vi "state_machine_aerial_robot_version_2.vi"() -> ()   [LabVIEW 2019]
uses:
  Control 1.ctl
  <vilib>/myRIO/Instrument Drivers/Onboard IO/DIO/typedefs/DIO Reference.ctl
  <vilib>/myRIO/Common/Instrument Driver Framework/Utilities/typedefs/myRIO Generic Hardware Reference.ctl
  <vilib>/myRIO/Common/Instrument Driver Framework/Utilities/typedefs/Hardware Version Enum.ctl
  <vilib>/myRIO/Common/Instrument Driver Framework/Utilities/typedefs/myRIO v1.0 Reference.ctl
  <vilib>/myRIO/Common/Instrument Driver Framework/Utilities/typedefs/Generic FPGA Reference.ctl
  <vilib>/myRIO/Common/Instrument Driver Framework/myRIO v1.0/DIO/typedefs/DIO Channels List.ctl
  <vilib>/myRIO/Common/Instrument Driver Framework/myRIO v1.0/DIO/typedefs/DIO Channels Enum.ctl
  <vilib>/userdefined/High Color/nirio_resource_hc.ctl
  <vilib>/myRIO/Common/Instrument Driver Framework/Utilities/vis/Is FPGA Ref Available.vi
  <vilib>/myRIO/Common/Instrument Driver Framework/myRIO v1.0/DIO/vis/myRIO v1.1 Open DIO.vi
  <vilib>/myRIO/Instrument Drivers/Onboard IO/DIO/vis/Write.vi
  <vilib>/myRIO/Common/Instrument Driver Framework/Utilities/vis/Validate Channels.vi
  <vilib>/myRIO/Common/Instrument Driver Framework/myRIO v1.0/DIO/vis/myRIO v1.0 Reserve DIO.vi
  <vilib>/myRIO/Common/Instrument Driver Framework/myRIO v1.0/Resource Manager/vis/myRIO v1.0 Reserve Channel List.vi
  <vilib>/myRIO/Common/Instrument Driver Framework/myRIO v1.0/DIO/vis/myRIO v1.0 Build MUX Configuration DIO.vi
  <vilib>/myRIO/Common/Instrument Driver Framework/myRIO v1.0/Resource Manager/vis/myRIO v1.0 Reserve Channel.vi
  <vilib>/myRIO/Common/Instrument Driver Framework/myRIO v1.0/Resource Manager/vis/myRIO v1.0 Unreserve Channel.vi
  <vilib>/myRIO/Common/Instrument Driver Framework/myRIO v1.0/Resource Manager/vis/myRIO v1.0 Create Configuration List.vi
  <vilib>/myRIO/Common/Instrument Driver Framework/myRIO v1.0/Resource Manager/vis/myRIO v1.0 Build Mutex Name.vi
  <vilib>/Utility/VariantDataType/GetNumericInfo.vi
  <vilib>/Utility/error.llb/Error Cluster From Error Code.vi
  <vilib>/myRIO/Common/Instrument Driver Framework/myRIO v1.0/myRIO v1.1 Open.vi
  <vilib>/myRIO/Common/Instrument Driver Framework/Utilities/vis/IO Manager.vi
  <vilib>/myRIO/Common/Instrument Driver Framework/Utilities/vis/Configuration Manager.vi
  <vilib>/myRIO/Common/Instrument Driver Framework/myRIO v1.0/Resource Manager/vis/myRIO v1.0 Configure IO.vi
  <vilib>/myRIO/Common/Instrument Driver Framework/myRIO v1.0/myRIO v1.0 Close.vi
  <vilib>/myRIO/Common/Instrument Driver Framework/myRIO v1.0/DIO/vis/myRIO v1.0 Write DIO.vi
  <vilib>/myRIO/Express VI/Onboard IO/DO/DO Express VI.xnode
  <vilib>/myRIO/Instrument Drivers/Onboard IO/DIO/vis/myRIO DIO Open.xnode
  <vilib>/myRIO/Express VI/Onboard Devices/LED/LED Express VI.xnode
  <vilib>/myRIO/Instrument Drivers/Onboard IO/DIO/DIO.lvlib
panel:
  out "Sensor_inserted?":bool
  out "drone_lifting?":bool
  out "measurement_number":i32
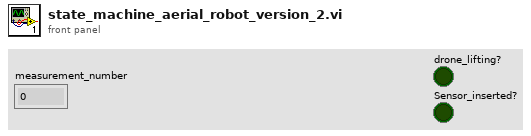
[diagram p1: front panel]
types:
  T1 = typedef "Control 1.ctl" = enum16{"Default", "state 1", "state 2", "state 3", "state 4", "state 5"}
  T2 = typedef "DIO.lvlib/DIO Reference.ctl" = cluster{"myRIO Reference":T3, "DIO Channels List":T7}
  T3 = typedef "myRIO Generic Hardware Reference.ctl" = cluster{"myRIO Model":T4, "myRIO Hardware Reference":T5}
  T4 = typedef "Hardware Version Enum.ctl" = enum16{"Unknown", "myRIO-1900", "myRIO-1950", "roboRIO", "NI ELVIS RIO CM", "ELVIS III"}
  T5 = typedef "myRIO v1.0 Reference.ctl" = cluster{"Generic FPGA Reference":T6, "Allow multiple opens":bool}
  T6 = typedef "Generic FPGA Reference.ctl" = refnum<k20>
  T7 = typedef "DIO Channels List.ctl" = T8[]
  T8 = typedef "DIO Channels Enum.ctl" = enum16{"Not Connected", "C/DIO0", "C/DIO1", "C/DIO2", "C/DIO3", "C/DIO4", "C/DIO5", "C/DIO6", "C/DIO7", "A/DIO0", "A/DIO1", "A/DIO2", "A/DIO3", "A/DIO4", "A/DIO5", "A/DIO6", "A/DIO7", "A/DIO8", "A/DIO9", "A/DIO10", "A/DIO11", "A/DIO12", "A/DIO13", "A/DIO14", "A/DIO15", "A/DIO16", "A/DIO17", "A/DIO18", "A/DIO19", "B/DIO0", "B/DIO1", "B/DIO2", "B/DIO3", "B/DIO4", "B/DIO5", "B/DIO6", "B/DIO7", "B/DIO8", "B/DIO9", "B/DIO10", "B/DIO11", "B/DIO12", "B/DIO13", "B/DIO14", "B/DIO15", "B/DIO16", "B/DIO17", "B/DIO18", "B/DIO19", "LED0", "LED1", "LED2", "LED3", "Button0", "DIO/DIO0", "DIO/DIO1", "DIO/DIO2", "DIO/DIO3", "DIO/DIO4", "DIO/DIO5", "DIO/DIO6", "DIO/DIO7", "DIO/DIO8", "DIO/DIO9", "SPI/CS0", "SPI/CS1", "SPI/CS2", "SPI/CS3", "LED RADIO (Green)", "LED RADIO (Red)", "LED COMM (Green)", "LED COMM (Red)", "LED MODE (Green)", "LED MODE (Red)"}
  T9 = typedef "nirio_resource_hc.ctl" = tag
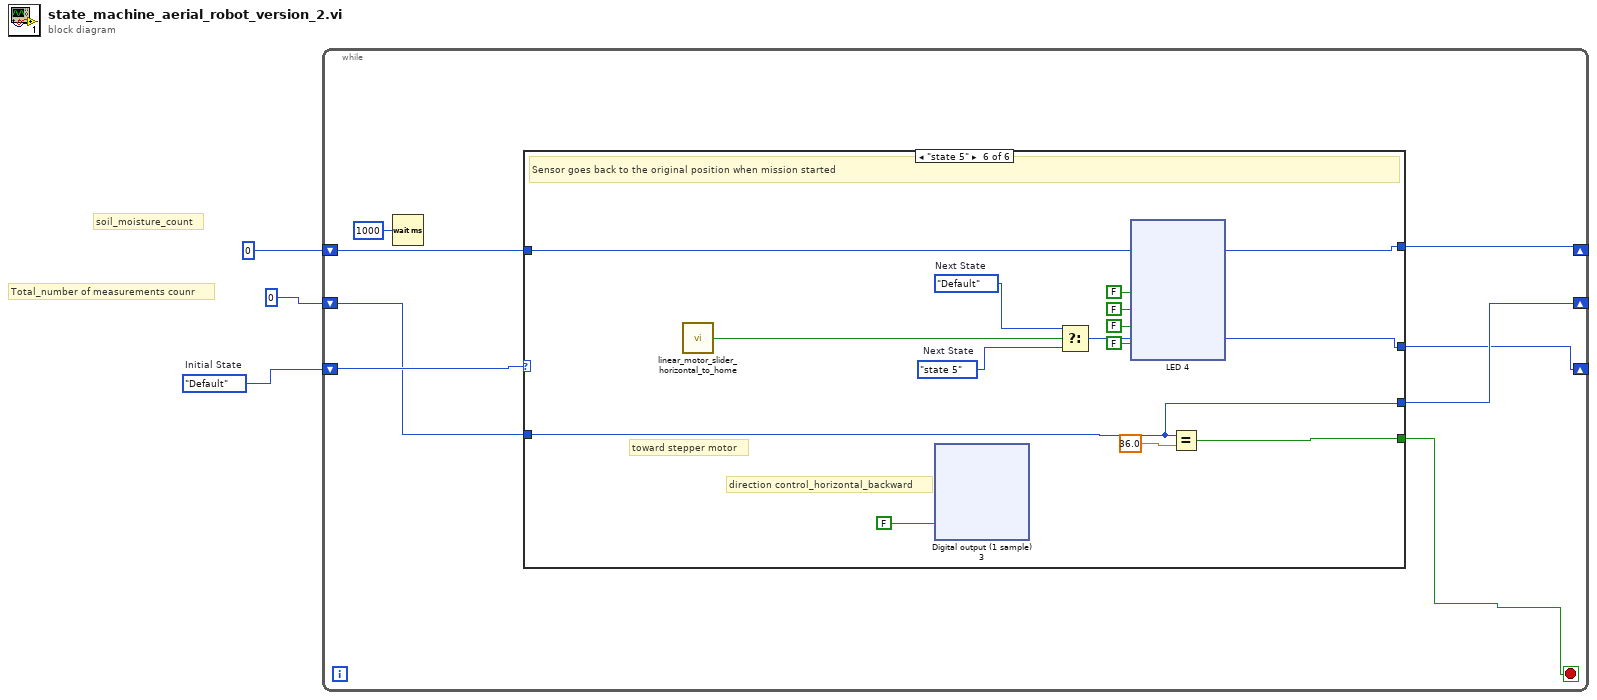
[diagram p0: block diagram]
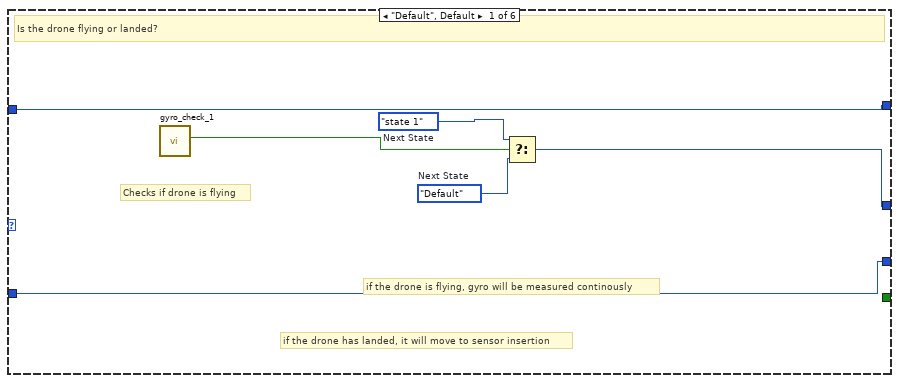
[diagram p2: hidden frame]
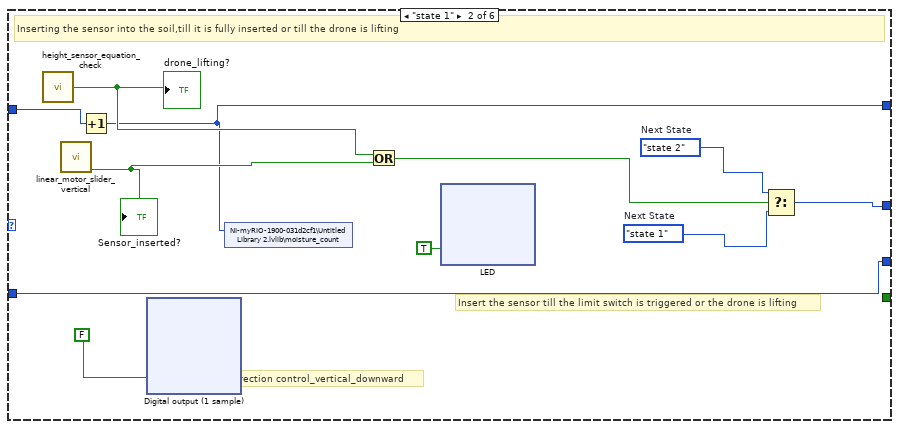
[diagram p3: hidden frame]
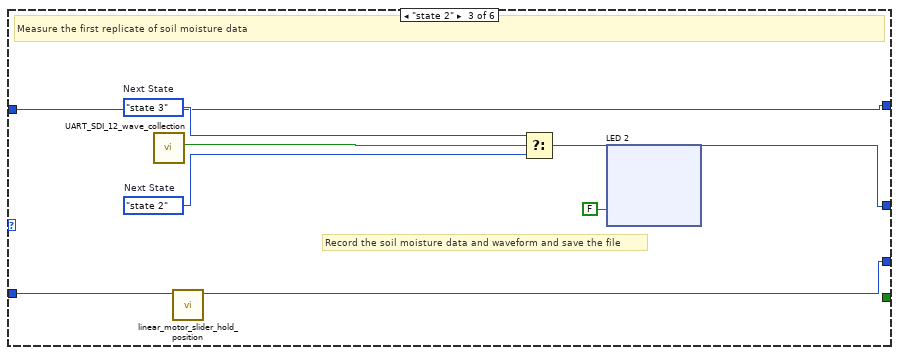
[diagram p4: hidden frame]
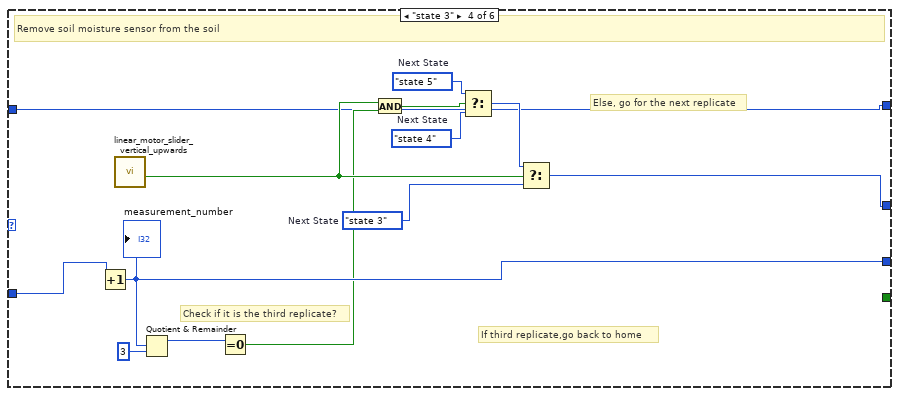
[diagram p5: hidden frame]
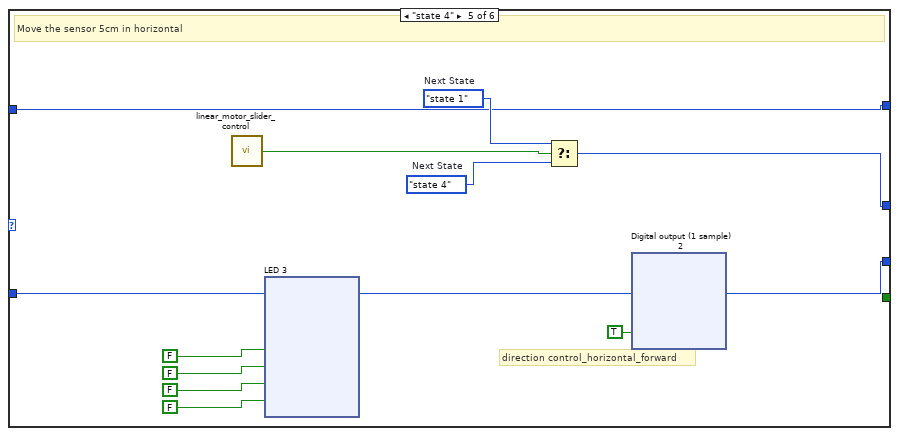
[diagram p6: hidden frame]
diagram:
  w3 = Control_1."Default"  # Initial State
  # "Total_number of measurements counr"
  # "soil_moisture_count"
  n1 = while {
    shift-right: [w9] -> _
    shift-left: 0 -> [w8]
    shift-right: [w7] -> _
    shift-left: w3 -> [w11]
    shift-right: [w5] -> _
    shift-left: 0 -> [w6]
    stop <- w4 stop-if-true
    n2 = Wait (ms)(milliseconds to wait=u32 1000) -> ()  [unwired: 1 out]
    n3 = case shown="\"state 5\"" w11 {
      tunnel: [w16 w28 w102 w152 w160 w248] -> w7
      tunnel: w8 -> [w13 w21 w101 w149 w159 w244]
      tunnel: [w13 w21 w101 w148 w159 w244] -> w9
      tunnel: [_ _ _ _ _ w243] -> w4
      tunnel: w6 -> [w12 w20 w100 w141 w158 w242]
      tunnel: [w12 w19 w100 w141 w158 w242] -> w5
      frame "Default", Default {
        w14 = Control_1."state 1"  # Next State
        w17 = Control_1."Default"  # Next State
        # "if the drone has landed, it will move to sensor insertion"
        # "if the drone is flying, gyro will be measured continously"
        # "Checks if drone is flying"
        # "Is the drone flying or landed?"
        n4 = call "gyro_check_1.vi"() -> ("has the drone landed?"=w15:bool)  [unwired: 11 in]
        n5 = Select(t=w14, s=w15, f=w17) -> (s? t:f=w16:T1)
      }
      frame "state 1" {
        w24 = Control_1."state 2"  # Next State
        w25 = Control_1."state 1"  # Next State
        # "Insert the sensor till the limit switch is triggered or the drone is lifting"
        # "direction control_vertical_downward"
        # "Inserting the sensor into the soil,till it is fully inserted or till the drone is lifting"
        n6 = call "height_sensor_equation_check.vi"() -> ("drone_lifting?"=w22:bool)  [unwired: 14 in, 1 out]
        "drone_lifting?" <- w22
        n7 = call "linear_motor_slider_vertical.vi"() -> ("Sensor_inserted?"=w23:bool)  [unwired: 11 in]
        "Sensor_inserted?" <- w23
        n8 = Increment(x=w20) -> (x+1=w19:i32)
        n9 = xnode "Digital output (1 sample)"("A/DIO10 (Pin 31)"=FALSE) -> ()  [unwired: 1 in, 1 out]
        n10 = shared-variable "NI-myRIO-1900-031d2cf1\\Untitled Library 2.lvlib\\moisture_count"(w19) -> ()  [unwired: 1 in, 1 out]
        n11 = Or(x=w22, y=w23) -> (x .or. y?=w27:bool)
        n12 = xnode "LED"("LED2"=TRUE) -> ()  [unwired: 1 in, 1 out]
        n13 = Select(t=w24, s=w27, f=w25) -> (s? t:f=w28:T1)
      }
      frame "state 2" {
        w104 = Control_1."state 3"  # Next State
        w105 = Control_1."state 2"  # Next State
        # "Record the soil moisture data and waveform and save the file"
        # "Measure the first replicate of soil moisture data"
        n14 = call "UART_SDI_12_wave_collection.vi"() -> ("soil moisture saved"=w103:bool)  [unwired: 11 in]
        n15 = call "linear_motor_slider_hold_position.vi"() -> ()  [unwired: 12 in]
        n16 = Select(t=w104, s=w103, f=w105) -> (s? t:f=w102:T1)
        n17 = xnode "LED 2"("LED2"=FALSE) -> ()  [unwired: 1 in, 1 out]
      }
      frame "state 3" {
        w143 = Control_1."state 5"  # Next State
        w144 = Control_1."state 4"  # Next State
        w153 = Control_1."state 3"  # Next State
        # "If third replicate,go back to home"
        # "Else, go for the next replicate"
        # "Check if it is the third replicate?"
        # "Remove soil moisture sensor from the soil"
        n18 = Increment(x=w149) -> (x+1=w148:i32)
        "measurement_number" <- w148
        n19 = call "linear_motor_slider_vertical_upwards.vi"() -> ("Reached desried steps"=w147:bool)  [unwired: 11 in]
        n20 = Quotient & Remainder(x=w148, y=3) -> (x-y*floor(x/y)=w150:i32)  [unwired: 1 out]
        n21 = Equal To 0?(x=w150) -> (x = 0?=w146:bool)
        n22 = And(x=w147, y=w146) -> (x .and. y?=w145:bool)
        n23 = Select(t=w143, s=w145, f=w144) -> (s? t:f=w142:T1)
        n24 = Select(t=w142, s=w147, f=w153) -> (s? t:f=w152:T1)
      }
      frame "state 4" {
        w163 = Control_1."state 1"  # Next State
        w164 = Control_1."state 4"  # Next State
        # "direction control_horizontal_forward"
        # "Move the sensor 5cm in horizontal"
        n25 = call "linear_motor_slider_control.vi"() -> ("5 cm reached?"=w162:bool)  [unwired: 11 in]
        n26 = xnode "LED 3"("LED0"=FALSE, "LED1"=FALSE, "LED2"=FALSE, "LED3"=FALSE) -> ()  [unwired: 1 in, 1 out]
        n27 = Select(t=w163, s=w162, f=w164) -> (s? t:f=w160:T1)
        n28 = xnode "Digital output (1 sample) 2"("B/DIO10 (Pin 31)"=TRUE) -> ()  [unwired: 1 in, 1 out]
      }
      frame "state 5" {
        w249 = Control_1."Default"  # Next State
        w250 = Control_1."state 5"  # Next State
        # "toward stepper motor"
        # "direction control_horizontal_backward"
        # "Sensor goes back to the original position when mission started"
        n29 = call "linear_motor_slider_horizontal_to_home.vi"() -> ("back to home?"=w247:bool)  [unwired: 11 in]
        n30 = xnode "Digital output (1 sample) 3"("B/DIO10 (Pin 31)"=FALSE) -> ()  [unwired: 1 in, 1 out]
        n31 = Select(t=w249, s=w247, f=w250) -> (s? t:f=w248:T1)
        n32 = xnode "LED 4"("LED0"=FALSE, "LED1"=FALSE, "LED2"=FALSE, "LED3"=FALSE) -> ()  [unwired: 1 in, 1 out]
        n33 = Equal?(x=w244, y=36.0) -> (x = y?=w243:bool)
      }
    }
  }
